vi "Generate Command Frame Vectors.vi"(0 "RFFE Command in":refnum<class "RFFE Command.lvclass">, 11 "error in (no error)":errorcluster) -> (4 "RFFE Command out":refnum<class "RFFE Command.lvclass">, 6 "Command Frame Vectors":string[](array[string]), 15 "error out":errorcluster)   [LabVIEW 2018, in "MIPI RFFE API.lvlib" / "RFFE Command.lvclass"]
uses:
  RFFE Command.lvclass
  RFFE Command.lvclass/RFFE Command.ctl
  Get Slave Address.vi
  Get Command Bits.vi
  MIPI RFFE API.lvlib
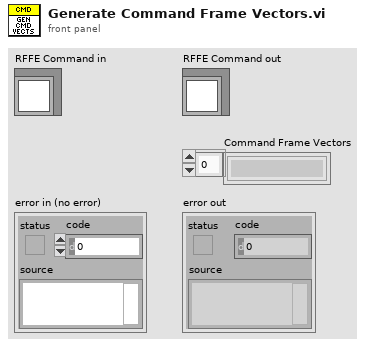
[diagram p1: front panel]
types:
  T1 = typedef "MIPI RFFE API.lvlib/Slave Address.ctl" = u8
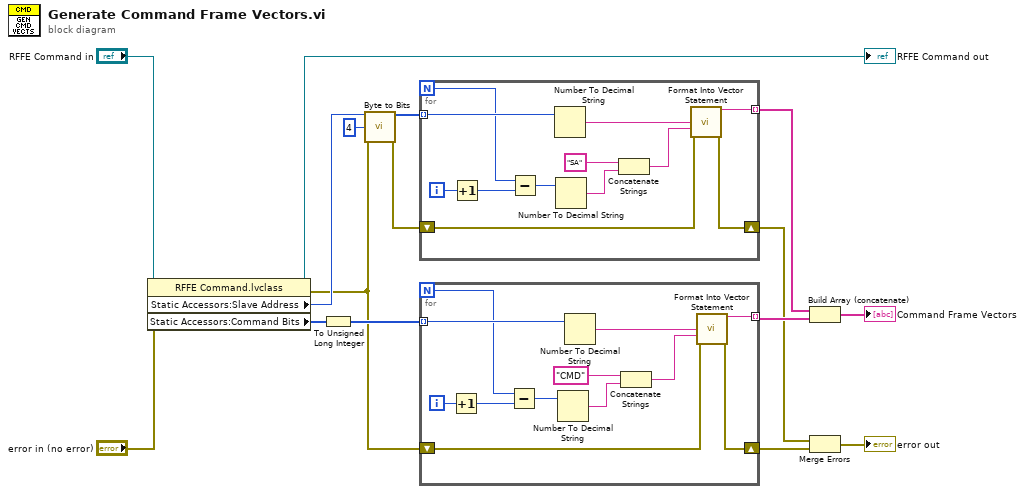
[diagram p0: block diagram]
diagram:
  n1 = property class="RFFE Command.lvclass"(reference="RFFE Command in", error in="error in (no error)") -> (reference out=→"RFFE Command out":refnum<class "RFFE Command.lvclass">, error out=w5:errorcluster, "Static Accessors:Slave Address"=w9:T1, "Static Accessors:Command Bits"=w11:u8[])
  n2 = To Unsigned Long Integer(number=w11) -> (unsigned 32bit integer=w10:u32[])
  n3 = call "Byte to Bits.vi"("Byte"=w9, "Bit Width"=4, "error in (no error)"=w5) -> ("Bits"=w7:u8[], "error out"=w6:errorcluster)  [unwired: 11 in]
  n4 = for {
    N -> [w21]
    tunnel: w7 -> [w28] mode=indexing
    shift-right: [w27] -> w1
    shift-left: w6 -> [w26]
    tunnel: [w17] -> w3 mode=indexing
    i -> [w20]
    n5 = Increment(x=w20) -> (x+1=w22:i32)
    n6 = Subtract(x=w21, y=w22) -> (x-y=w19:i32)
    n7 = Number To Decimal String(number=w28) -> (decimal integer string=w25:string)  [unwired: 1 in]
    n8 = Number To Decimal String(number=w19) -> (decimal integer string=w23:string)  [unwired: 1 in]
    n9 = Concatenate Strings("SA" ("string"), w23) -> (w18:string)
    n10 = call "Format Into Vector Statement.vi"("DATA (0)"=w25, "Comment"=w18, "error in (no error)"=w26) -> ("Vector Statement"=w17:string, "error out"=w27:errorcluster)  [unwired: 11 in]
  }
  n11 = for {
    N -> [w31]
    shift-right: [w38] -> w2
    shift-left: w5 -> [w39]
    tunnel: [w37] -> w4 mode=indexing
    tunnel: w10 -> [w36] mode=indexing
    i -> [w32]
    n12 = Increment(x=w32) -> (x+1=w30:i32)
    n13 = Subtract(x=w31, y=w30) -> (x-y=w29:i32)
    n14 = Number To Decimal String(number=w29) -> (decimal integer string=w35:string)  [unwired: 1 in]
    n15 = Number To Decimal String(number=w36) -> (decimal integer string=w40:string)  [unwired: 1 in]
    n16 = Concatenate Strings("CMD" ("string"), w35) -> (w33:string)
    n17 = call "Format Into Vector Statement.vi"("DATA (0)"=w40, "Comment"=w33, "error in (no error)"=w39) -> ("Vector Statement"=w37:string, "error out"=w38:errorcluster)  [unwired: 11 in]
  }
  n18 = Build Array (concatenate)(w3, w4) -> (→"Command Frame Vectors":string[])
  n19 = Merge Errors(w1, w2) -> (→"error out":errorcluster)
